vi "CRYAdd rep #s to data headers.vi"(11 "Data array in":T1 {"Z data" items=["dB", "Lin"]; "X data" items=["dB", "Lin"]; "Y data" items=["dB", "Lin"]; "Z dB ref" format="%.1f"; "Z axis" items=["Log", "Lin"]; "X dB ref" format="%.1f"; "X axis" items=["Log", "Lin"]; "Y axis" items=["Log", "Lin"]; "Y dB ref" format="%.1f"; "Curve"."z" format="%.2f"; "Curve"."y" format="%.2f"; "Curve"."x" format="%.2f"}) -> (3 "Data array with rep #'s":T1 {"Z data" items=["dB", "Lin"]; "X data" items=["dB", "Lin"]; "Y data" items=["dB", "Lin"]; "Z dB ref" format="%.1f"; "Z axis" items=["Log", "Lin"]; "X dB ref" format="%.1f"; "X axis" items=["Log", "Lin"]; "Y axis" items=["Log", "Lin"]; "Y dB ref" format="%.1f"; "Curve"."z" format="%.2f"; "Curve"."y" format="%.2f"; "Curve"."x" format="%.2f"})   [LabVIEW 2013]
uses:
  Typedef Control/CRYData Cluster Array.ctl
  Typedef Control/CRYData Cluster.ctl
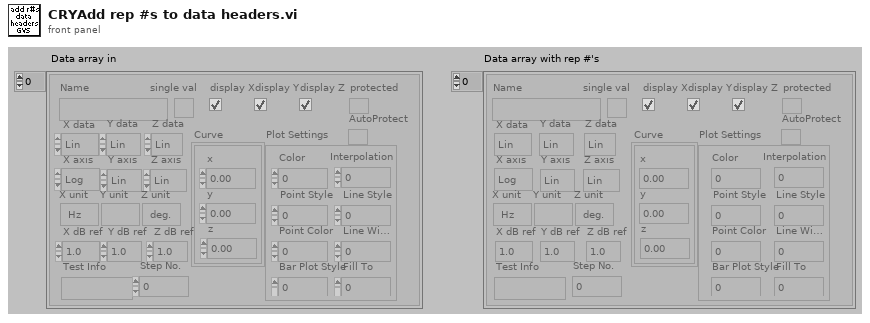
[diagram p1: front panel]
types:
  T1 = typedef "CRYData Cluster Array.ctl" = T2[]
  T2 = typedef "CRYData Cluster.ctl" = cluster{"Name":string, "Curve":cluster{"x":dbl, "y":dbl, "z":dbl}[], "X data":u16, "Y data":u16, "Z data":u16, "X axis":u16, "Y axis":u16, "Z axis":u16, "X unit":string, "Y unit":string, "Z unit":string, "X dB ref":dbl, "Y dB ref":dbl, "Z dB ref":dbl, "single val":bool, "protected":bool, "display X":bool, "display Y":bool, "display Z":bool, "Test Info":string, "Step No.":i32, "Plot Settings":cluster{"Color":u32, "Interpolation":u8, "Point Style":u8, "Line Style":u8, "Point Color":u32, "Line Width":u8, "Bar Plot Style":u8, "Fill To":i16}, "AutoProtect":bool}
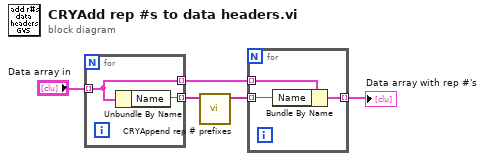
[diagram p0: block diagram]
diagram:
  n1 = for {
    tunnel: [w7] -> w5 mode=indexing
    tunnel: [w6] -> w3 mode=indexing
    tunnel: "Data array in" -> [w6] mode=indexing
    n2 = Unbundle By Name(w6) -> ("Name"=w7:string)
  }
  n3 = call "CRYAppend rep # prefixes.vi"("Curves list in"=w5) -> ("Curves list with no repeats"=w4:string[])  [unwired: 10 out]
  n4 = for {
    tunnel: w4 -> [w9] mode=indexing
    tunnel: w3 -> [w10] mode=indexing
    tunnel: [w8] -> w1 mode=indexing
    n5 = Bundle By Name(cluster=w10, "Name"=w9) -> (w8:T2)
  }
  "Data array with rep #'s" <- w1
